vi "SlideCoincidence.vi"(3 "shift (photons)":u32, 4 "lateral peaks":u32, 5 "window (photons)":u32, 6 "center peak (µs)":dbl format="%.2f", 7 "delay channel":i32, 8 "histogram lenght (µs)":dbl format="%.2f", 9 "rawdata":T1) -> (0 "SlideTime":dbl[](array[numeric]) format="%.2f", 1 "SlideCoincidence":dbl[](array[numeric]) format="%.2f", 2 "SlideCenterPeak":u32[](array[numeric]))   [LabVIEW 2009]
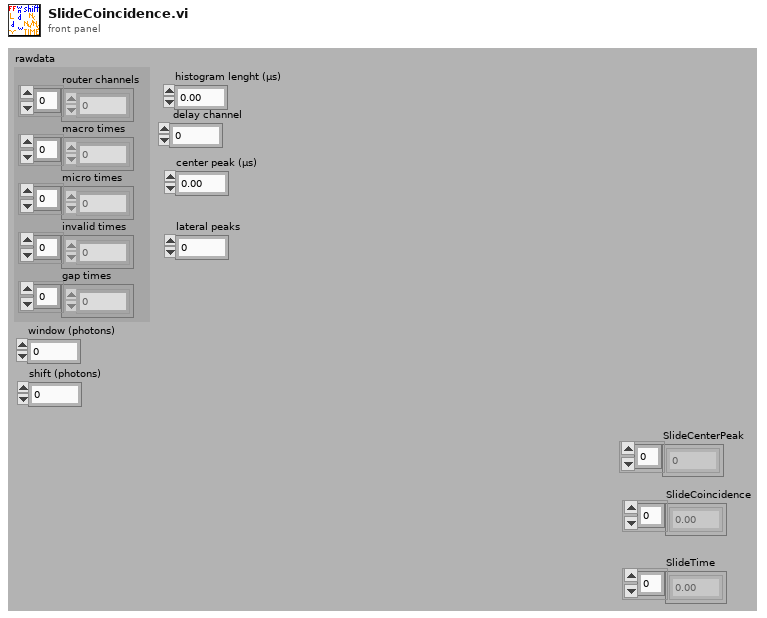
[diagram p1: front panel]
types:
  T1 = cluster{"router channels":u8[], "macro times":u32[], "micro times":u16[], "invalid times":u32[], "gap times":u32[]}
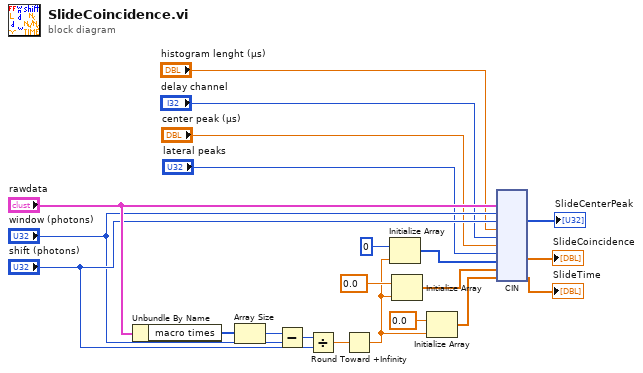
[diagram p0: block diagram]
diagram:
  n1 = Unbundle By Name("rawdata") -> ("macro times"=w19:u32[])
  n2 = Array Size(array=w19) -> (size(s)=w18:i32)
  n3 = Subtract(x=w18, y="window (photons)") -> (x-y=w17:u32)
  n4 = Divide(x=w17, y="shift (photons)") -> (x/y=w15:dbl)
  n5 = Round Toward +Infinity(x=w15) -> (ceil(x): smallest int >= x=w2:dbl)
  n6 = Initialize Array(u32 0 ("element"), w2) -> (w3:u32[])
  n7 = Initialize Array(0.0 ("element"), w2) -> (w11:dbl[])
  n8 = Initialize Array(0.0 ("element"), w2) -> (w13:dbl[])
  n9 = cin ("Code Interface Node")("rawdata", "window (photons)", "shift (photons)", "histogram lenght (µs)", "delay channel", "center peak (µs)", "lateral peaks", w3, w11, w13) -> (→"SlideCenterPeak":u32[], →"SlideCoincidence":dbl[], →"SlideTime":dbl[])  [unwired: 7 in]
